vi "Create Message Data Cluster.vi"(7 "Owning vi ref (typeDef)":refnum<vi>, 8 "error in (no error)":errorcluster, 10 "Message Elements MetaData":T1[](array[typedef]), 11 "Cluster ref in":refnum<vi>) -> (0 "error out":errorcluster, 3 "Cluster ref out":refnum<vi>)   [LabVIEW 2019, in "gRPC Scripting Tools.lvlib"]
uses:
  gRPC Scripting Tools.lvlib
  TypeDefs/Message Element Metadata (Scripting).ctl
  TypeDefs/Message Element Type.ctl
  <vilib>/Utility/miscctls.llb/LVPositionTypeDef.ctl
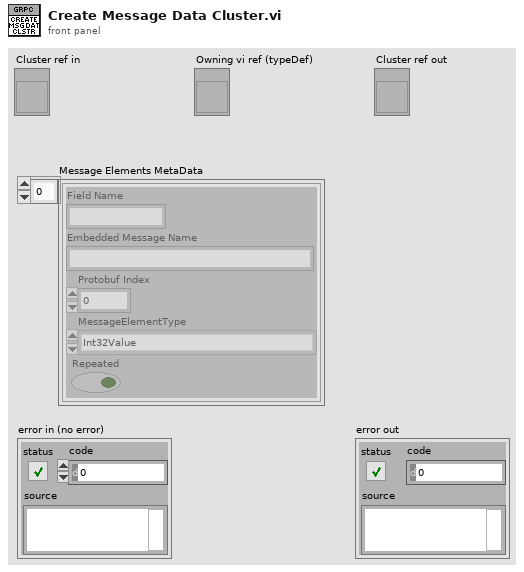
[diagram p1: front panel]
types:
  T1 = typedef "gRPC Scripting Tools.lvlib/Message Element Metadata (Scripting).ctl" = cluster{"Field Name":string, "Embedded Message Name":string, "Protobuf Index":i32, "MessageElementType":T2, "Repeated":bool}
  T2 = typedef "gRPC Scripting Tools.lvlib/Message Element Type.ctl" = enum32{"Int32Value", "FloatValue", "DoubleValue", "BoolValue", "StringValue", "MessageValue", "Int64Value", "UInt32Value", "UInt64Value", "EnumValue"}
  T3 = typedef "LVPositionTypeDef.ctl" = cluster{"Left":i32, "Top":i32}
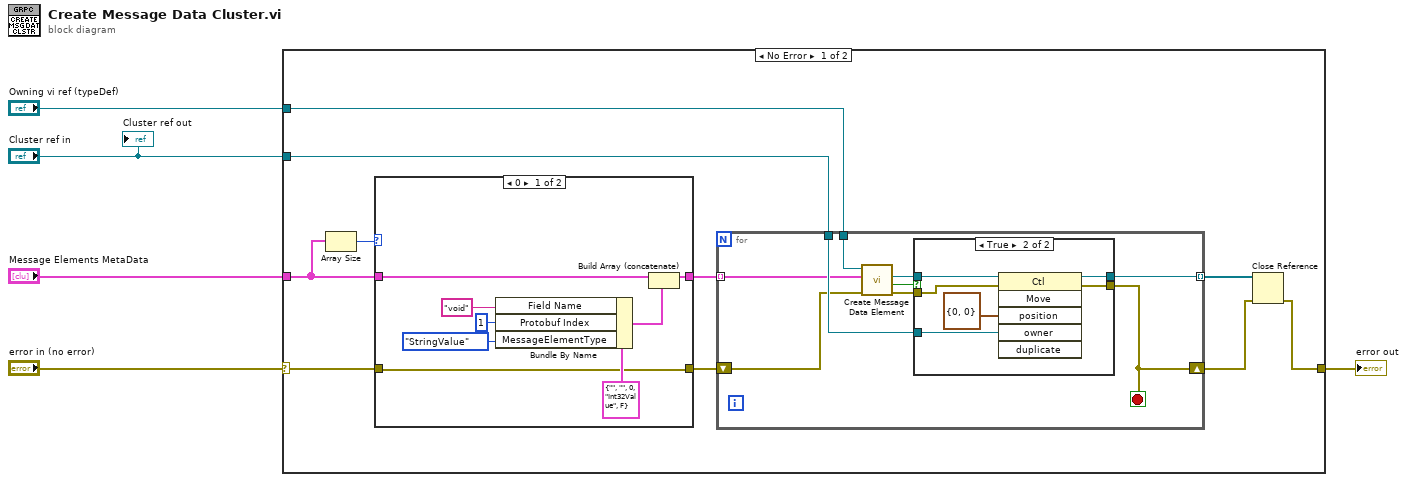
[diagram p0: block diagram]
diagram:
  n1 = case shown="No Error" "error in (no error)" {
    selector: "error in (no error)" -> [w7 w43]
    tunnel: "Message Elements MetaData" -> [w9 _]
    tunnel: [w14 w43] -> w4
    tunnel: "Cluster ref in" -> [w13 _]
    tunnel: "Owning vi ref (typeDef)" -> [w12 _]
    frame No Error {
      n2 = Array Size(array=w9) -> (size(s)=w10:i32)
      n3 = case shown="0" w10 {
        tunnel: w9 -> [w23 w24]
        tunnel: [w22 w24] -> w8
        tunnel: w7 -> [w16 w25]
        tunnel: [w16 w25] -> w6
        frame 0 {
          n4 = Bundle By Name(cluster=T1 {"Field Name"="", "Embedded Message Name"="", "Protobuf Index"=0, "MessageElementType"=enum."Int32Value", "Repeated"=FALSE} ("MessageElementMetadata"), "Field Name"="void", "Protobuf Index"=1, "MessageElementType"=Message_Element_Type."StringValue") -> (w17:T1)
          n5 = Build Array (concatenate)(w23, w17) -> (w22:T1[])
        }
        frame 1, Default {
        }
      }
      n6 = for {
        tunnel: w13 -> [w34]
        tunnel: [w33] -> w15 mode=indexing
        tunnel: w12 -> [w32]
        shift-right: [w28] -> w11
        shift-left: w6 -> [w29]
        tunnel: w8 -> [w26] mode=indexing
        stop <- w28 stop-if-true
        n7 = call "Create Message Data Element.vi"("error in (no error)"=w29, "Message Element MetaData"=w26, "Owning vi in"=w32) -> ("error out"=w30:errorcluster, "Data Element Created"=w27:bool, "Data Element ref out (Ctrl ref)"=w31:refnum<vi>)  [unwired: 5 in, 1 out]
        n8 = case shown="True" w27 {
          tunnel: w34 -> [_ w42]
          tunnel: [w36 w41] -> w33
          tunnel: w31 -> [w36 w39]
          tunnel: w30 -> [w35 w38]
          tunnel: [w35 w37] -> w28
          frame False {
          }
          frame True {
            n9 = invoke class="Ctl" method="Move"(reference=w39, error in=w38, "position"=T3 {"Left"=0, "Top"=0}, "owner"=w42) -> (reference out=w41:refnum<vi>, error out=w37:errorcluster)  [unwired: 2 in, 4 out]
          }
        }
      }
      n10 = Close Reference(reference=w15, error in (no error)=w11) -> (error out=w14:errorcluster)
    }
    frame Error {
    }
  }
  "error out" <- w4
  "Cluster ref out" <- "Cluster ref in"
